vi "Test Multitone.vi"() -> ()   [LabVIEW 2016, in "Lockin.DAQ.lvclass"]
uses:
  Lockin.DAQ.lvclass
  <vilib>/measure/NI_MAPro.lvlib
  <vilib>/measure/NI_MABase.lvlib
panel:
  out "timer 3 (ms)":u32
  out "timer 2 (ms)":u32
  out "timer 1 (ms)":u32
  out "Waveform Graph":waveform(dbl)[](graph)
  out "resulting string":string
  in  "phase":dbl[](array[numeric])
  in  "frequency":dbl[](array[numeric])
  in  "amplitude":dbl[](array[numeric])
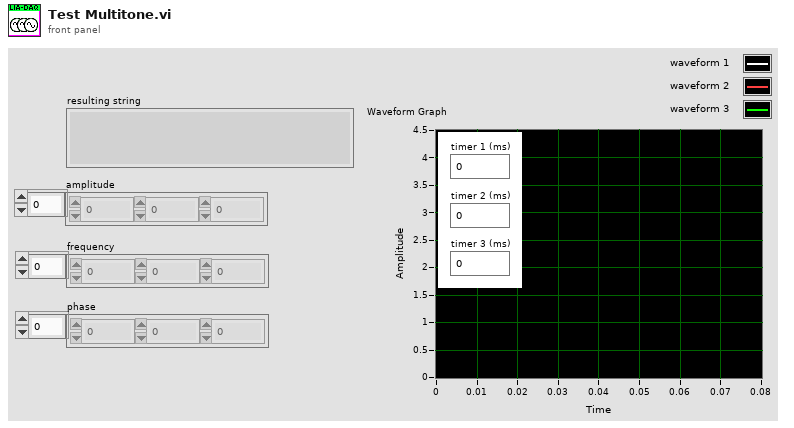
[diagram p1: front panel]
types:
  T1 = enum16{"Sine Wave", "Triangle Wave", "Square Wave", "Sawtooth Wave"}
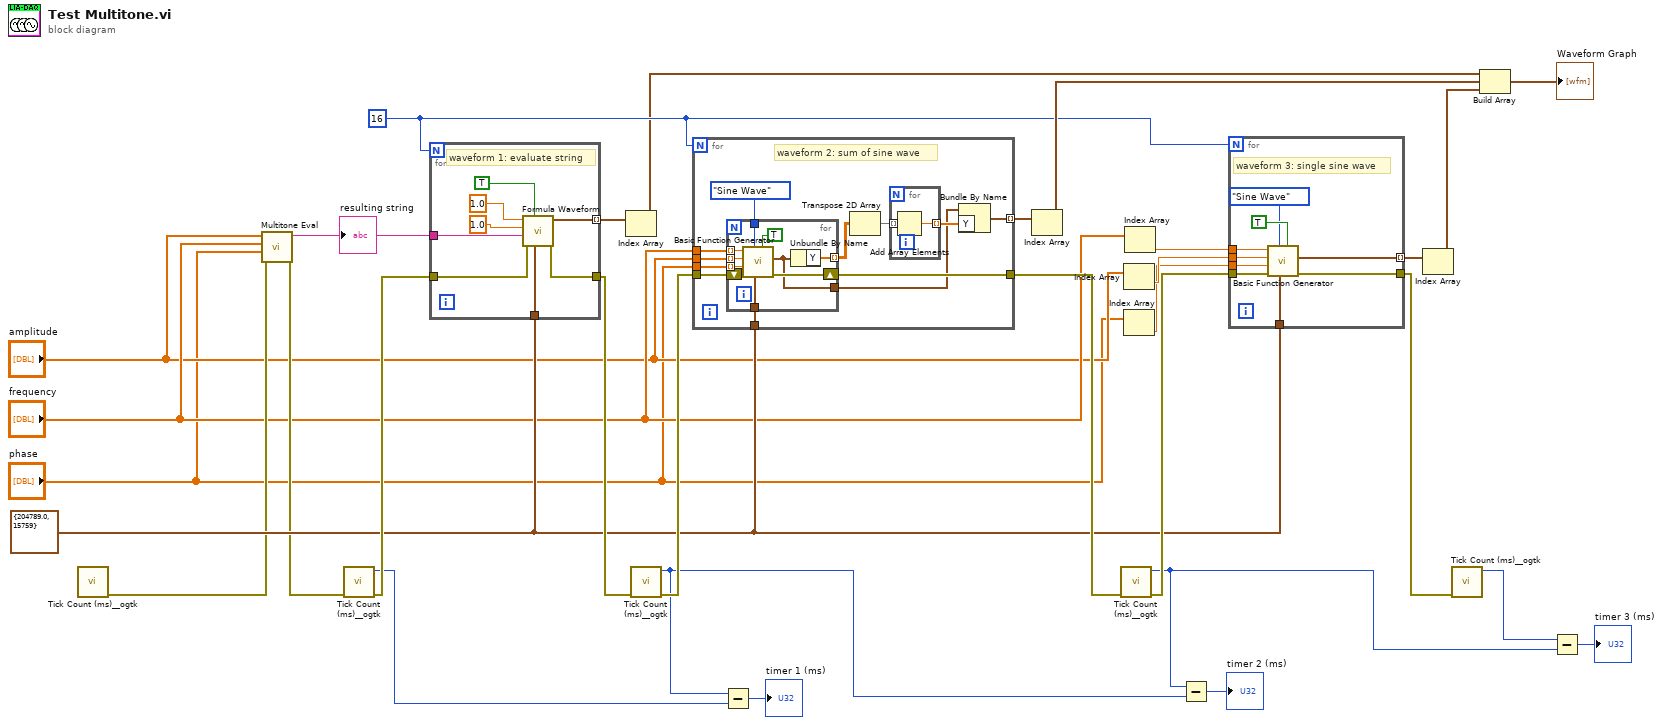
[diagram p0: block diagram]
diagram:
  w6 = 16
  w26 = cluster{"Fs":dbl, "#s":i32} {"Fs"=204789.0, "#s"=15759} ("sampling")
  n1 = call <userlib>:"Tick Count (ms)__ogtk.vi"() -> ("error out"=w24:errorcluster)  [unwired: 10 in, 1 out]
  n2 = call "Multitone Eval.vi"("error in (no error)"=w24, "phase"="phase", "frequency"="frequency", "amplitude"="amplitude") -> ("error out"=w23:errorcluster, "String"=w22:string)  [unwired: 6 in]
  "resulting string" <- w22
  n3 = call <userlib>:"Tick Count (ms)__ogtk.vi"("error in (no error)"=w23) -> ("error out"=w31:errorcluster, "millisecond timer value"=w14:u32)  [unwired: 9 in]
  n4 = for {
    N: w6 -> [_]
    tunnel: w26 -> [w39]
    tunnel: w22 -> [w38]
    tunnel: w31 -> [w34]
    tunnel: [w33] -> w30
    tunnel: [w32] -> w21 mode=indexing
    # "waveform 1: evaluate string"
    n5 = call <vilib>:"Formula Waveform.vi"("sampling info"=w39, "reset signal"=TRUE, "error in (no error)"=w34, "formula"=w38, "amplitude"=1.0, "frequency"=1.0) -> ("error out"=w33:errorcluster, "signal out"=w32:waveform(dbl))  [unwired: 4 in]
  }
  n6 = Index Array(array=w21) -> (element=w2:waveform(dbl))  [unwired: 1 in]
  n7 = call <userlib>:"Tick Count (ms)__ogtk.vi"("error in (no error)"=w30) -> ("error out"=w29:errorcluster, "millisecond timer value"=w3:u32)  [unwired: 9 in]
  n8 = for {
    N: w6 -> [_]
    tunnel: w29 -> [w51]
    tunnel: w26 -> [w50]
    tunnel: [w49] -> w28
    tunnel: "frequency" -> [w48]
    tunnel: "amplitude" -> [w47]
    tunnel: "phase" -> [w46]
    tunnel: [w43] -> w16 mode=indexing
    # "waveform 2: sum of sine wave"
    n9 = for {
      tunnel: w50 -> [w62]
      shift-right: [w61] -> w49
      shift-left: w51 -> [w63]
      tunnel: w48 -> [w60] mode=indexing
      tunnel: w47 -> [w59] mode=indexing
      tunnel: w46 -> [w58] mode=indexing
      tunnel: T1."Sine Wave" ("signal type") -> [w57]
      tunnel: [w56] -> w40 mode=indexing
      tunnel: [w55] -> w41
      n10 = call <vilib>:"Basic Function Generator.vi"("reset signal"=TRUE, "sampling info"=w62, "signal type"=w57, "error in (no error)"=w63, "phase"=w58, "amplitude"=w59, "frequency"=w60) -> ("error out"=w61:errorcluster, "signal out"=w55:waveform(dbl))  [unwired: 2 in, 1 out]
      n11 = Unbundle By Name(w55) -> ("Y"=w56:dbl[])
    }
    n12 = Transpose 2D Array(2D array=w40) -> (transposed array=w44:dbl[][])
    n13 = for {
      tunnel: w44 -> [w53] mode=indexing
      tunnel: [w52] -> w42 mode=indexing
      n14 = Add Array Elements(numeric array=w53) -> (sum=w52:dbl)
    }
    n15 = Bundle By Name(cluster=w41, "Y"=w42) -> (w43:waveform(dbl))
  }
  n16 = Subtract(x=w3, y=w14) -> (x-y=→"timer 1 (ms)":u32)
  n17 = Index Array(array=w16) -> (element=w8:waveform(dbl))  [unwired: 1 in]
  n18 = call <userlib>:"Tick Count (ms)__ogtk.vi"("error in (no error)"=w28) -> ("error out"=w27:errorcluster, "millisecond timer value"=w12:u32)  [unwired: 9 in]
  n19 = Index Array(array="amplitude") -> (element=w5:dbl)  [unwired: 1 in]
  n20 = Index Array(array="phase") -> (element=w4:dbl)  [unwired: 1 in]
  n21 = Index Array(array="frequency") -> (element=w19:dbl)  [unwired: 1 in]
  n22 = Subtract(x=w12, y=w3) -> (x-y=→"timer 2 (ms)":u32)
  n23 = for {
    N: w6 -> [_]
    tunnel: w27 -> [w72]
    tunnel: w26 -> [w71]
    tunnel: [w70] -> w25
    tunnel: w19 -> [w69]
    tunnel: [w66] -> w15 mode=indexing
    tunnel: w5 -> [w65]
    tunnel: w4 -> [w64]
    # "waveform 3: single sine wave"
    n24 = call <vilib>:"Basic Function Generator.vi"("reset signal"=TRUE, "sampling info"=w71, "signal type"=T1."Sine Wave", "error in (no error)"=w72, "phase"=w64, "amplitude"=w65, "frequency"=w69) -> ("error out"=w70:errorcluster, "signal out"=w66:waveform(dbl))  [unwired: 2 in, 1 out]
  }
  n25 = Index Array(array=w15) -> (element=w1:waveform(dbl))  [unwired: 1 in]
  n26 = call <userlib>:"Tick Count (ms)__ogtk.vi"("error in (no error)"=w25) -> ("millisecond timer value"=w13:u32)  [unwired: 9 in, 1 out]
  n27 = Build Array(w2, w8, w1) -> (→"Waveform Graph":waveform(dbl)[])
  n28 = Subtract(x=w13, y=w12) -> (x-y=→"timer 3 (ms)":u32)
